vi "sign.vi"(0 "HGF_GPG":refnum<class "HGF_GPG.lvclass">, 1 "options file":path, 2 "keyringfile":path, 3 "Sec keyringfile":path, 4 "string in":string, 5 "error in (no error)":errorcluster, 6 "key-id":string, 7 "password":string, 8 "Trust DB":path) -> (10 "dup Trust DB":path, 11 "success":bool=TRUE, 13 "data error":bool, 14 "dup HGF_GPG":refnum<class "HGF_GPG.lvclass">, 15 "dup options file":path, 16 "dup keyringfile":path, 17 "dup Sec keyringfile":path, 18 "String out":string, 19 "error out":errorcluster)   [LabVIEW 2012, in "HGF_GPG.lvlib" / "HGF_GPG.lvclass"]
doc: "Sign a string."
uses:
  HGF_GPG.lvclass
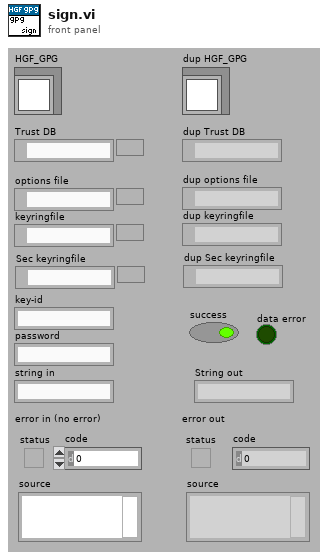
[diagram p1: front panel]
types:
  T1 = enum16{"open", "replace", "create", "open or create", "replace or create", "replace or create with confirmation"}
  T2 = enum16{"encrypt", "decrypt", "sign", "verify", "sign & encrypt", "verify & decrypt"}
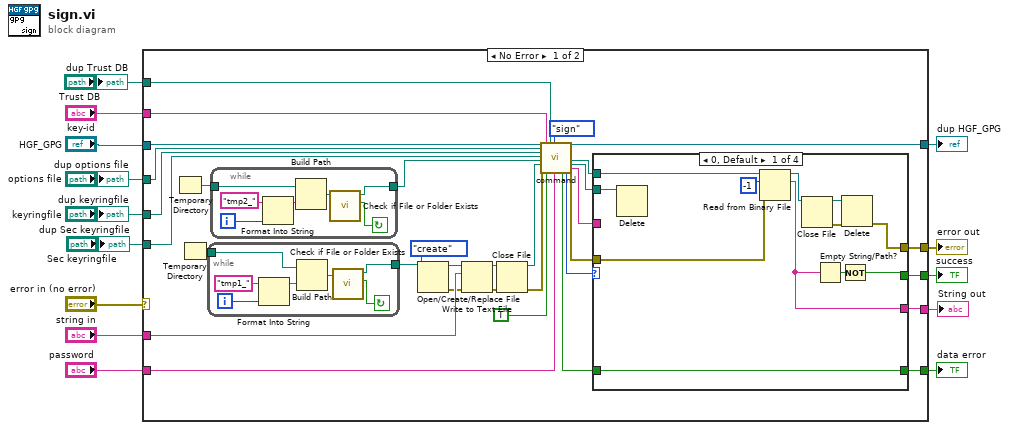
[diagram p0: block diagram]
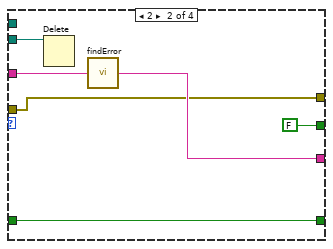
[diagram p2: hidden frame]
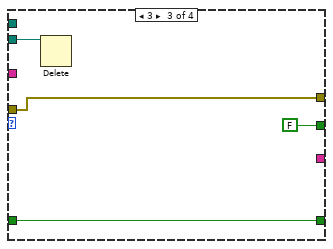
[diagram p3: hidden frame]
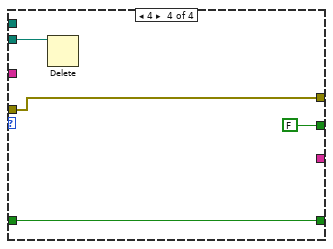
[diagram p4: hidden frame]
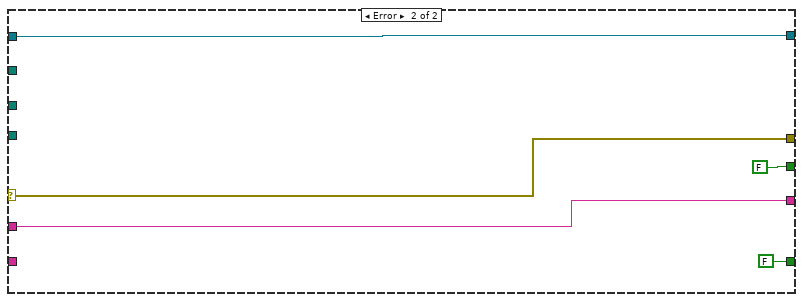
[diagram p5: hidden frame]
diagram:
  n1 = case shown="No Error" "error in (no error)" {
    selector: "error in (no error)" -> [_ w90]
    tunnel: [w45 w91] -> w12
    tunnel: "HGF_GPG" -> [w46 w91]
    tunnel: [w39 w90] -> w9
    tunnel: "string in" -> [w44 w89]
    tunnel: [w38 w89] -> w10
    tunnel: [w31 FALSE ("data error?")] -> w8
    tunnel: [w30 FALSE] -> w7
    tunnel: "password" -> [w23 _]
    tunnel: "key-id" -> [w17 _]
    tunnel: "options file" -> [w27 _]
    tunnel: "keyringfile" -> [w26 _]
    tunnel: "Sec keyringfile" -> [w16 _]
    tunnel: "Trust DB" -> [w15 _]
    frame No Error {
      n2 = Temporary Directory() -> (w33:path)
      n3 = Temporary Directory() -> (w34:path)
      n4 = while {
        tunnel: [w86] -> w37
        tunnel: w34 -> [w84]
        i -> [w82]
        stop <- w85 continue-if-true
        n5 = Format Into String(initial string="tmp1_" ("name or relative path"), w82) -> (resulting string=w81:string)  [unwired: 2 in, 1 out]
        n6 = Build Path(base path=w84, name or relative path=w81) -> (appended path=w80:path)
        n7 = call <vilib>:"Check if File or Folder Exists.vi"("path"=w80) -> ("file or folder exists?"=w85:bool, "dup path"=w86:path)  [unwired: 1 in, 8 out]
      }
      n8 = while {
        tunnel: w33 -> [w79]
        tunnel: [w77] -> w25
        i -> [w75]
        stop <- w76 continue-if-true
        n9 = Format Into String(initial string="tmp2_" ("name or relative path"), w75) -> (resulting string=w74:string)  [unwired: 2 in, 1 out]
        n10 = Build Path(base path=w79, name or relative path=w74) -> (appended path=w78:path)
        n11 = call <vilib>:"Check if File or Folder Exists.vi"("path"=w78) -> ("file or folder exists?"=w76:bool, "dup path"=w77:path)  [unwired: 1 in, 8 out]
      }
      n12 = Open/Create/Replace File(file path (use dialog)=w37, operation (0:open)=T1."create") -> (refnum out=w36:refnum<file>, error out=w32:errorcluster)  [unwired: 1 in, 4 out]
      n13 = Write to Text File(file (use dialog)=w36, text=w44, error in=w32) -> (refnum out=w43:refnum<file>, error out=w42:errorcluster)  [unwired: 2 out]
      n14 = Close File(refnum=w43, error in=w42) -> (path=w24:path, error out=w41:errorcluster)
      n15 = call-dynamic "command.vi"("HGF_GPG"=w46, "options file"=w27, "keyringfile"=w26, "Sec keyringfile"=w16, "targetfile"=w25, "sourcefile"=w24, "error in (no error)"=w41, "key-id"=w17, "overwrite? (t)"=TRUE ("overwrite?"), "Trust DB"=w15, "task"=T2."sign", "password"=w23) -> ("data error"=w40:bool, "return code"=w18:i32, "dup HGF_GPG"=w45:refnum<class "HGF_GPG.lvclass">, "dup targetfile"=w22:path, "dup sourcefile"=w21:path, "standard error"=w20:string, "error out"=w19:errorcluster)  [unwired: 1 in, 8 out]
      n16 = case shown="0, Default" w18 {
        tunnel: w20 -> [_ w62 _ _]
        tunnel: w19 -> [w47 w63 w68 w72]
        tunnel: w40 -> [w53 w59 w65 w69]
        tunnel: [w56 w63 w68 w72] -> w39
        tunnel: [w52 w64 _ _] -> w38
        tunnel: [w53 w59 w65 w69] -> w31
        tunnel: [w50 FALSE FALSE FALSE] -> w30
        tunnel: w22 -> [w49 _ _ _]
        tunnel: w21 -> [w48 w60 w66 w70]
        frame 0, Default {
          n17 = Delete(path (use dialog)=w48) -> ()  [unwired: 1 in, 6 out]
          n18 = Read from Binary File(8:w47, 10:-1 ("count (1)"), 11:w49) -> (2:w52:string, 3:w58:refnum<file>)  [unwired: 5 out]
          n19 = Close File(refnum=w58) -> (path=w55:path, error out=w57:errorcluster)  [unwired: 1 in]
          n20 = Empty String/Path?(string/path=w52) -> (empty?=w51:bool)
          n21 = Not(x=w51) -> (.not. x?=w50:bool)
          n22 = Delete(path (use dialog)=w55, error in=w57) -> (error out=w56:errorcluster)  [unwired: 5 out]
        }
        frame 2 {
          n23 = Delete(path (use dialog)=w60) -> ()  [unwired: 1 in, 6 out]
          n24 = call "findError.vi"("error string in"=w62) -> ("error out"=w64:string)
        }
        frame 3 {
          n25 = Delete(path (use dialog)=w66) -> ()  [unwired: 1 in, 6 out]
        }
        frame 4 {
          n26 = Delete(path (use dialog)=w70) -> ()  [unwired: 1 in, 6 out]
        }
      }
    }
    frame Error {
    }
  }
  "error out" <- w9
  "dup HGF_GPG" <- w12
  "String out" <- w10
  "success" <- w7
  "data error" <- w8
  "dup options file" <- "options file"
  "dup keyringfile" <- "keyringfile"
  "dup Sec keyringfile" <- "Sec keyringfile"
  "dup Trust DB" <- "Trust DB"
